vi "ic6_logic_statement.vi"(1 "Logic statement":string[](array[string])) -> (0 "Byte output":u8[](array[numeric]))   [LabVIEW 2012]
uses:
  <vilib>/Utility/file.llb/Read From Spreadsheet File (string).vi
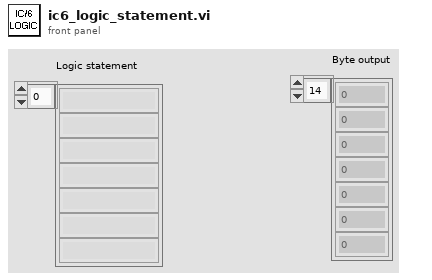
[diagram p1: front panel]
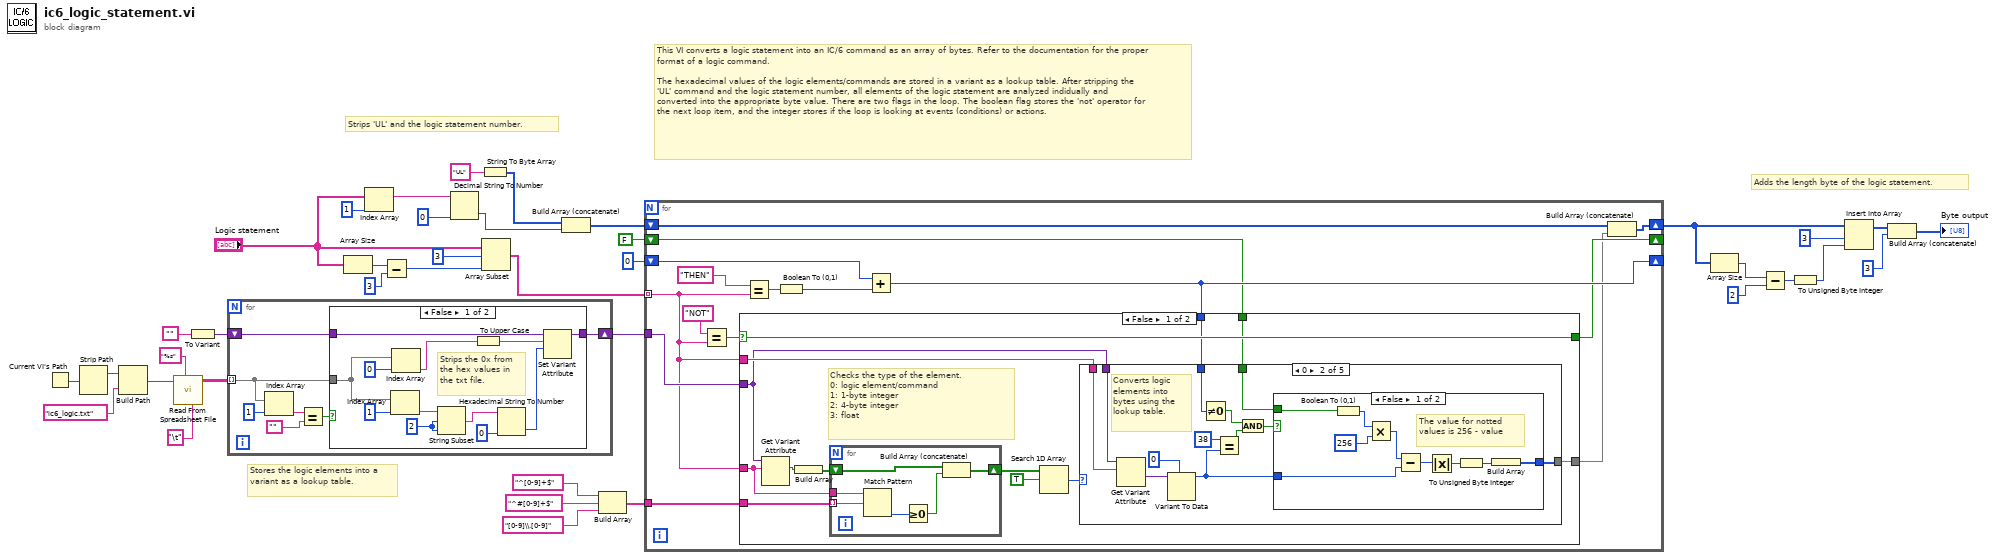
[diagram p0: block diagram]
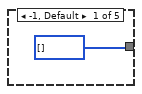
[diagram p2: hidden frame]
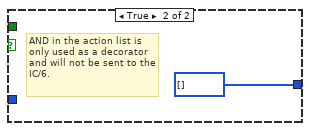
[diagram p3: hidden frame]
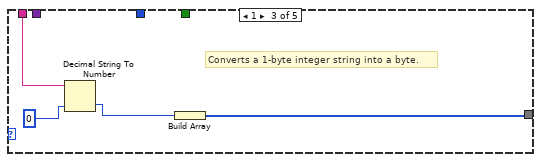
[diagram p4: hidden frame]
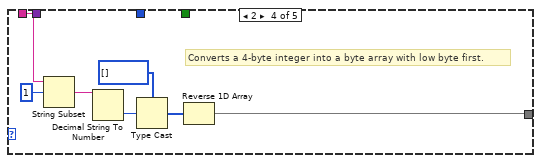
[diagram p5: hidden frame]
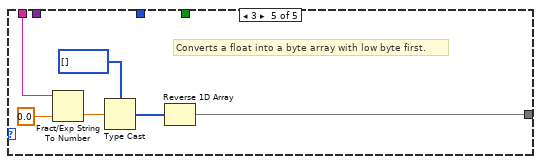
[diagram p6: hidden frame]
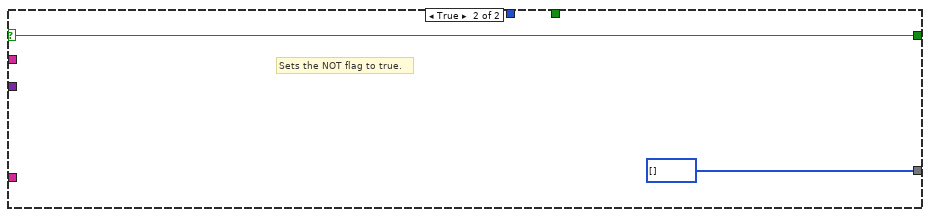
[diagram p7: hidden frame]
diagram:
  # "Adds the length byte of the logic statement."
  # "Stores the logic elements into a variant as a lookup table."
  # "Strips 'UL' and the logic statement number."
  # "This VI converts a logic statement into an IC/6 command as an array of bytes. Refer to the documentation for the proper format of a logic command. \n\nThe hexadecimal values of the logic elements/commands are stored in a variant as a lookup table. After stripping the 'UL' command and the logic statement number, all elements of the logic statement are analyzed indidually and converted into the appropriate byte value. There are two flags in the loop. The boolean flag stores the 'not' operator for the next loop item, and the integer stores if the loop is looking at events (conditions) or actions."
  n1 = Current VI's Path() -> (path=w38:path)
  n2 = Strip Path(path=w38) -> (stripped path=w37:path)  [unwired: 1 out]
  n3 = Build Path(base path=w37, name or relative path="ic6_logic.txt") -> (appended path=w30:path)
  n4 = call-poly <vilib>:"Read From Spreadsheet File.vi"("delimiter (\\t)"="\t", "format (%s)"="%s", "file path (dialog if empty)"=w30) -> ("all rows"=w33:string[][])  [unwired: 4 in, 4 out]
  n5 = To Variant(anything="") -> (Variant=w31:variant)
  n6 = for {
    tunnel: w33 -> [w41] mode=indexing
    shift-right: [w39] -> w29
    shift-left: w31 -> [w40]
    n7 = Index Array(array=w41, index=1) -> (element=w44:string)
    n8 = Equal?(x=w44, y="") -> (x = y?=w42:bool)
    n9 = case shown="False" w42 {
      tunnel: w41 -> [w54 _]
      tunnel: w40 -> [w51 w58]
      tunnel: [w50 w58] -> w39
      frame False {
        w56 = 2
        # "Strips the 0x from the hex values in the txt file."
        n10 = Index Array(array=w54, index=1) -> (element=w57:string)
        n11 = Index Array(array=w54, index=0) -> (element=w52:string)
        n12 = String Subset(string=w57, offset (0)=w56, length (rest)=w56) -> (substring=w48:string)
        n13 = To Upper Case(1:w52) -> (0:w46:string)
        n14 = Hexadecimal String To Number(string=w48, default (0uL)=0) -> (number=w49:i32)  [unwired: 1 in, 1 out]
        n15 = Set Variant Attribute(Variant=w51, name=w46, value=w49) -> (Variant out=w50:variant)  [unwired: 1 in, 2 out]
      }
      frame True {
        # "The condition is true for lines without tab character, i.e. blank lines and decorators."
      }
    }
  }
  n16 = Array Size(array="Logic statement") -> (size(s)=w21:i32)
  n17 = Index Array(array="Logic statement", index=1) -> (element=w14:string)
  n18 = Subtract(x=w21, y=3) -> (x-y=w12:i32)
  n19 = Decimal String To Number(string=w14, default (0L)=u8 0) -> (number=w17:u8)  [unwired: 1 in, 1 out]
  n20 = String To Byte Array(string="UL") -> (unsigned byte array=w15:u8[])
  n21 = Array Subset(array="Logic statement", index=3, length=w12) -> (w27:string[])
  n22 = Build Array (concatenate)(w15, w17) -> (w26:u8[])
  n23 = Build Array("^[0-9]+$", "^#[0-9]+$", "[0-9]\\.[0-9]") -> (w22:string[])
  n24 = for {
    tunnel: w27 -> [w59] mode=indexing
    shift-right: [w71] -> w5
    shift-left: w26 -> [w70]
    tunnel: w29 -> [w72]
    tunnel: w22 -> [w73]
    shift-right: [w64] -> _
    shift-left: i16 0 -> [w65]
    shift-right: [w61] -> _
    shift-left: FALSE -> [w62]
    n25 = Equal?(x="NOT", y=w59) -> (x = y?=w63:bool)
    n26 = Equal?(x="THEN", y=w59) -> (x = y?=w67:bool)
    n27 = Boolean To (0,1)(Boolean=w67) -> (0, 1=w66:i16)
    n28 = Add(x=w65, y=w66) -> (x+y=w64:i16)
    n29 = case shown="False" w63 {
      selector: w63 -> [w76 w133]
      tunnel: w73 -> [w83 _]
      tunnel: w59 -> [w82 _]
      tunnel: w72 -> [w77 _]
      tunnel: [w79 u8[] []] -> w60
      tunnel: w59 -> [w78 _]
      tunnel: w64 -> [w74 _]
      tunnel: w62 -> [w75 _]
      tunnel: [w76 w133] -> w61
      frame False {
        # "Checks the type of the element.\n0: logic element/command\n1: 1-byte integer\n2: 4-byte integer\n3: float"
        n30 = Get Variant Attribute(Variant=w77, name=w82) -> (found=w81:bool)  [unwired: 2 in, 3 out]
        n31 = Build Array(w81) -> (w80:bool[])
        n32 = for {
          tunnel: w82 -> [w132]
          shift-right: [w130] -> w84
          shift-left: w80 -> [w129]
          tunnel: w83 -> [w127] mode=indexing
          n33 = Match Pattern(string=w132, regular expression=w127) -> (offset past match=w128:i32)  [unwired: 1 in, 3 out]
          n34 = Greater Or Equal To 0?(x=w128) -> (x >= 0?=w131:bool)
          n35 = Build Array (concatenate)(w129, w131) -> (w130:bool[])
        }
        n36 = Search 1D Array(1D array=w84, element=TRUE) -> (index of element=w86:i32)  [unwired: 1 in]
        n37 = case shown="0" w86 {
          tunnel: [u8[] [] w97 w112 w115 w122] -> w79
          tunnel: w78 -> [_ w98 w110 w114 w121]
          tunnel: w77 -> [_ w99 _ _ _]
          tunnel: w74 -> [_ w89 _ _ _]
          tunnel: w75 -> [_ w88 _ _ _]
          frame -1, Default {
          }
          frame 0 {
            # "Converts logic elements into bytes using the lookup table."
            n38 = Get Variant Attribute(Variant=w99, name=w98) -> (value=w96:variant)  [unwired: 2 in, 3 out]
            n39 = Variant To Data(type=i16 0, Variant=w96) -> (data=w94:i16)  [unwired: 1 in, 1 out]
            n40 = Not Equal To 0?(x=w89) -> (x != 0?=w90:bool)
            n41 = Equal?(x=i16 38, y=w94) -> (x = y?=w92:bool)
            n42 = And(x=w90, y=w92) -> (x .and. y?=w91:bool)
            n43 = case shown="False" w91 {
              tunnel: [w108 u8[] []] -> w97
              tunnel: w94 -> [w104 _]
              tunnel: w88 -> [w100 _]
              frame False {
                # "The value for notted values is 256 - value"
                n44 = Boolean To (0,1)(Boolean=w100) -> (0, 1=w102:i16)
                n45 = Multiply(x=w102, y=i16 256) -> (x*y=w101:i16)
                n46 = Subtract(x=w101, y=w104) -> (x-y=w105:i16)
                n47 = Absolute Value(x=w105) -> (abs(x)=w106:i16)
                n48 = To Unsigned Byte Integer(number=w106) -> (unsigned 8bit integer=w107:u8)
                n49 = Build Array(w107) -> (w108:u8[])
              }
              frame True {
                # "AND in the action list is only used as a decorator and will not be sent to the IC/6."
              }
            }
          }
          frame 1 {
            # "Converts a 1-byte integer string into a byte."
            n50 = Decimal String To Number(string=w110, default (0L)=u8 0) -> (number=w111:u8)  [unwired: 1 in, 1 out]
            n51 = Build Array(w111) -> (w112:u8[])
          }
          frame 2 {
            # "Converts a 4-byte integer into a byte array with low byte first."
            n52 = String Subset(string=w114, offset (0)=1) -> (substring=w119:string)  [unwired: 1 in]
            n53 = Decimal String To Number(string=w119) -> (number=w118:i32)  [unwired: 2 in, 1 out]
            n54 = Type Cast(type=u8[] [], x=w118) -> (*(type *) &x=w116:u8[])
            n55 = Reverse 1D Array(array=w116) -> (reversed array=w115:u8[])
          }
          frame 3 {
            # "Converts a float into a byte array with low byte first."
            n56 = Fract/Exp String To Number(string=w121, default (0 dbl)=sgl 0.0) -> (number=w126:sgl)  [unwired: 2 in, 1 out]
            n57 = Type Cast(type=u8[] [], x=w126) -> (*(type *) &x=w125:u8[])
            n58 = Reverse 1D Array(array=w125) -> (reversed array=w122:u8[])
          }
        }
      }
      frame True {
        # "Sets the NOT flag to true."
      }
    }
    n59 = Build Array (concatenate)(w70, w60) -> (w71:u8[])
  }
  n60 = Array Size(array=w5) -> (size(s)=w10:i32)
  n61 = Subtract(x=w10, y=2) -> (x-y=w8:i32)
  n62 = To Unsigned Byte Integer(number=w8) -> (unsigned 8bit integer=w7:u8)
  n63 = Insert Into Array(array=w5, index=3, new element=w7) -> (w4:u8[])
  n64 = Build Array (concatenate)(w4, u8 3) -> (→"Byte output":u8[])
